vi "Test Increments.vi"() -> ()   [LabVIEW 2013]
uses:
  source/Time Increment Units -- enum.ctl
  source/Compare Timestamps.vi
  source/EpochNotTimestamp.vi
panel:
  out "1 minute - No DST 2":bool
  out "1 minute - With DST 2":bool
  out "ISO8601 UTC DateTime":string
  out "1 month - With DST":bool
  out "1 month - No DST":bool
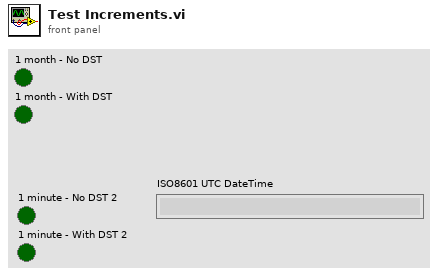
[diagram p1: front panel]
types:
  T1 = typedef "Time Increment Units -- enum.ctl" = enum16{"week", "day", "hour", "minute", "second", "millisecond", "microsecond", "nanosecond", "month", "year"}
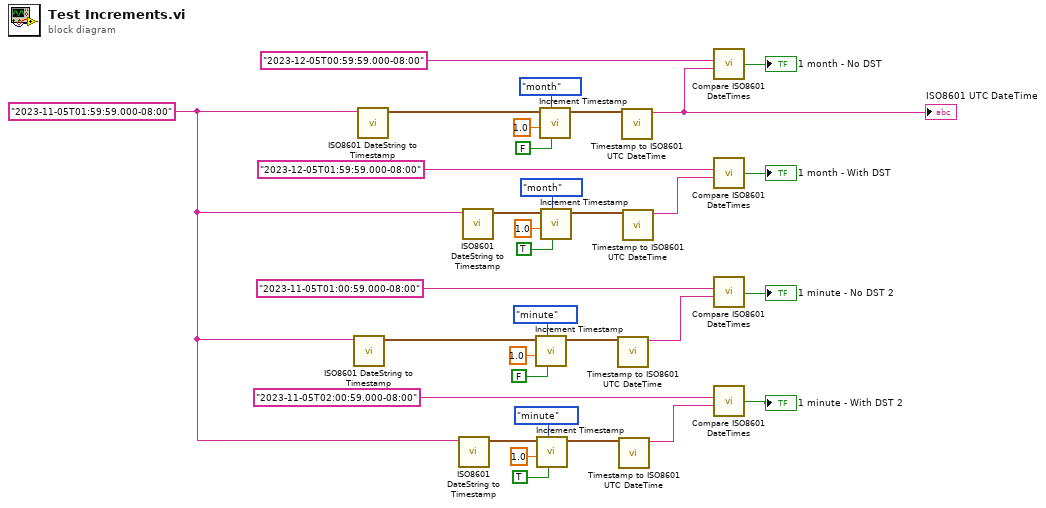
[diagram p0: block diagram]
diagram:
  w13 = "2023-11-05T01:59:59.000-08:00" ("ISO8601 UTC DateTime")
  n1 = call "ISO8601 DateString to Timestamp.vi"("ISO8601 Date String"=w13) -> ("Timestamp"=w23:timestamp)  [unwired: 8 in, 2 out]
  n2 = call "ISO8601 DateString to Timestamp.vi"("ISO8601 Date String"=w13) -> ("Timestamp"=w24:timestamp)  [unwired: 8 in, 2 out]
  n3 = call "ISO8601 DateString to Timestamp.vi"("ISO8601 Date String"=w13) -> ("Timestamp"=w22:timestamp)  [unwired: 8 in, 2 out]
  n4 = call "ISO8601 DateString to Timestamp.vi"("ISO8601 Date String"=w13) -> ("Timestamp"=w25:timestamp)  [unwired: 8 in, 2 out]
  n5 = call "Increment Timestamp.vi"("Account for DST?"=FALSE, "Unit (second)"=Time_Increment_Units_--_enum."minute", "Resolution (in selected unit)"=1.0, "timestamp (now)"=w23) -> ("timestamp"=w16:timestamp)  [unwired: 6 in]
  n6 = call "Increment Timestamp.vi"("Account for DST?"=TRUE, "Unit (second)"=Time_Increment_Units_--_enum."minute", "Resolution (in selected unit)"=1.0, "timestamp (now)"=w22) -> ("timestamp"=w19:timestamp)  [unwired: 6 in]
  n7 = call "Increment Timestamp.vi"("Account for DST?"=FALSE, "Unit (second)"=Time_Increment_Units_--_enum."month", "Resolution (in selected unit)"=1.0, "timestamp (now)"=w24) -> ("timestamp"=w31:timestamp)  [unwired: 6 in]
  n8 = call "Increment Timestamp.vi"("Account for DST?"=TRUE, "Unit (second)"=Time_Increment_Units_--_enum."month", "Resolution (in selected unit)"=1.0, "timestamp (now)"=w25) -> ("timestamp"=w28:timestamp)  [unwired: 6 in]
  n9 = call "Timestamp to ISO8601 UTC DateTime.vi"("Timestamp (now)"=w16) -> ("ISO8601 UTC DateTime"=w6:string)  [unwired: 10 in]
  n10 = call "Timestamp to ISO8601 UTC DateTime.vi"("Timestamp (now)"=w19) -> ("ISO8601 UTC DateTime"=w5:string)  [unwired: 10 in]
  n11 = call "Timestamp to ISO8601 UTC DateTime.vi"("Timestamp (now)"=w31) -> ("ISO8601 UTC DateTime"=w10:string)  [unwired: 10 in]
  "ISO8601 UTC DateTime" <- w10
  n12 = call "Timestamp to ISO8601 UTC DateTime.vi"("Timestamp (now)"=w28) -> ("ISO8601 UTC DateTime"=w8:string)  [unwired: 10 in]
  n13 = call "Compare ISO8601 DateTimes.vi"("ISO8601 DateTime (1)"="2023-12-05T00:59:59.000-08:00" ("ISO8601 UTC DateTime"), "ISO8601 DateTime (2)"=w10) -> ("Equal?"=→"1 month - No DST":bool)  [unwired: 6 in]
  n14 = call "Compare ISO8601 DateTimes.vi"("ISO8601 DateTime (1)"="2023-12-05T01:59:59.000-08:00" ("ISO8601 UTC DateTime"), "ISO8601 DateTime (2)"=w8) -> ("Equal?"=→"1 month - With DST":bool)  [unwired: 6 in]
  n15 = call "Compare ISO8601 DateTimes.vi"("ISO8601 DateTime (1)"="2023-11-05T01:00:59.000-08:00" ("ISO8601 UTC DateTime"), "ISO8601 DateTime (2)"=w6) -> ("Equal?"=→"1 minute - No DST 2":bool)  [unwired: 6 in]
  n16 = call "Compare ISO8601 DateTimes.vi"("ISO8601 DateTime (1)"="2023-11-05T02:00:59.000-08:00" ("ISO8601 UTC DateTime"), "ISO8601 DateTime (2)"=w5) -> ("Equal?"=→"1 minute - With DST 2":bool)  [unwired: 6 in]
